vi "Get StationGlobal.vi"() -> ()   [LabVIEW 2020]
uses:
  Engine/Get StationGlobals Prop.vi
  VariableContainer/VariableContainer.lvclass
  Engine/Engine.lvclass
panel:
  out "error out":errorcluster
  out "Original Value":string
  in  "Lookup String":string="Channel"
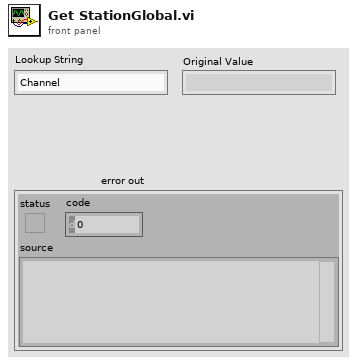
[diagram p1: front panel]
types:
  T1 = typedef "TSS.lvlib/Engine.lvclass/Session Handle.ctl" = refnum<data-value>
  T2 = typedef "TSS.lvlib/VariableContainer.lvclass/Session Handle.ctl" = refnum<data-value>
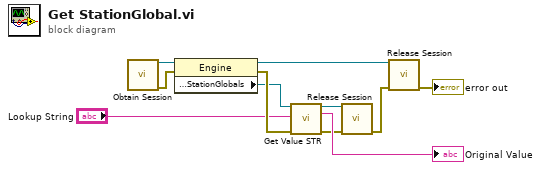
[diagram p0: block diagram]
diagram:
  n1 = call "Obtain Session.vi"() -> ("Session Handle"=w8:T1, "error out"=w10:errorcluster)  [unwired: 14 in]
  n2 = property class="Engine"(reference=w8, error in=w10) -> (reference out=w7:T1, error out=w9:errorcluster, "Properties:StationGlobals"=w6:T2)
  n3 = call "Get Value STR.vi"("Session Handle in"=w6, "Lookup String"="Lookup String", "error in (no error)"=w9) -> ("Session Handle out"=w3:T2, "Value"=→"Original Value":string, "error out"=w2:errorcluster)  [unwired: 9 in, 1 out]
  n4 = call "Release Session.vi"("Session Handle"=w3, "error in (no error)"=w2) -> ("error out"=w1:errorcluster)  [unwired: 13 in]
  n5 = call "Release Session.vi"("Session Handle"=w7, "error in (no error)"=w1) -> ("error out"=→"error out":errorcluster)  [unwired: 13 in]
